vi "Write Unit Label.vi"(5 "Unit Label":refnum<class "Text.lvclass">, 9 "Numeric in":refnum<class "Numeric.lvclass">) -> (3 "Numeric out":refnum<class "Numeric.lvclass">)   [LabVIEW 2014, in "Numeric.lvclass"]
uses:
  Numeric.lvclass
  Text/Text.lvclass
  Numeric.lvclass/Numeric.ctl
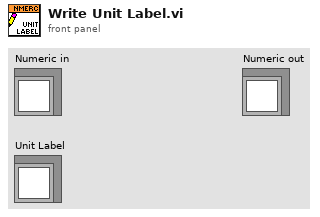
[diagram p1: front panel]
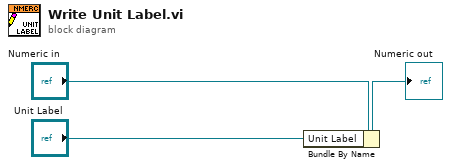
[diagram p0: block diagram]
diagram:
  n1 = Bundle By Name(cluster="Numeric in", "Unit Label"="Unit Label") -> (→"Numeric out":refnum<class "Numeric.lvclass">)
